vi "UltraDriver.vi"(7 "Port/MUX":T1={"Port"=3, "MUX Port"=0} {"Port" items=["Port 1", "Port 2", "Port 3", "Port 4"]; "MUX Port" items=["No MUX", "MUX 1", "MUX 2", "MUX 3", "MUX 4"]}, 11 "NXT In":T3 caption="NXT") -> (2 "Distance (cm)":i16, 3 "NXT Out":T3 caption="NXT")   [LabVIEW 2012]
uses:
  <vilib>/NXT/Subs/LVHSConnector.ctl
  <vilib>/NXT/LegoClasses/BrickReference/BrickReference.lvclass
  <vilib>/NXT/HiTechnic/HiTechnic Controls/HiTechnic Port.ctl
  <vilib>/NXT/Block Support/NXT_InputPort.ctl
  <vilib>/NXT/HiTechnic/HiTechnic LEGO MUX/HiTechnic Ultrasonic_cm MUX.vi
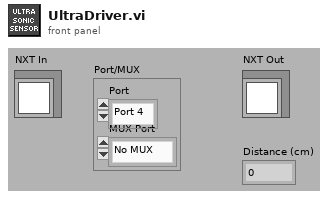
[diagram p1: front panel]
types:
  T1 = typedef "HiTechnic Port.ctl" = cluster{"Port":T2, "MUX Port":u8}
  T2 = typedef "NXT_InputPort.ctl" = u8
  T3 = typedef "LVHSConnector.ctl" = refnum<class "BrickReference.lvclass">
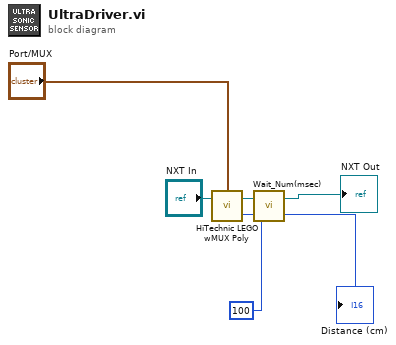
[diagram p0: block diagram]
diagram:
  n1 = call-poly <vilib>:"HiTechnic LEGO wMUX Poly.vi"("NXT"="NXT In", "Port/MUX"="Port/MUX") -> ("Distance (cm)"=→"Distance (cm)":i16, "NXT"=w5:T3)  [unwired: 1 in]
  n2 = call <vilib>:"Wait_Num(msec).vi"("Time (100 msec)"=u32 100, "NXT"=w5) -> ("NXT"=→"NXT Out":T3)  [unwired: 2 in]
